vi "Motic Get Temperature.vi"(8 "error in (no error)":errorcluster, 11 "camera":i32) -> (0 "error out":errorcluster, 1 "ambient temperature out":sgl, 2 "sensor surface temperature out":sgl, 3 "camera out":i32, 4 "relative humidity out":sgl, 5 "is temperature data available?":bool)   [LabVIEW 2012, in "MoticApi.lvlib"]
doc: "MOTICAPI bool Motic_GetTemperature(MUCam_Handle camera, float* st, float*at, float*rh);"
uses:
  MoticApi.lvlib
  MoticApi.dll
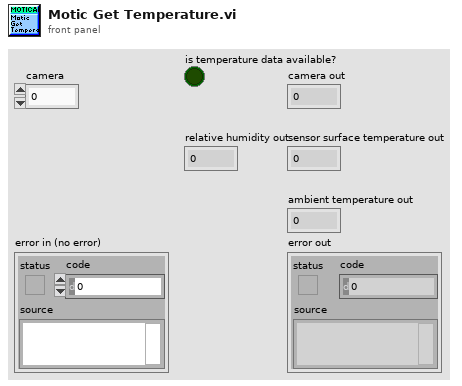
[diagram p1: front panel]
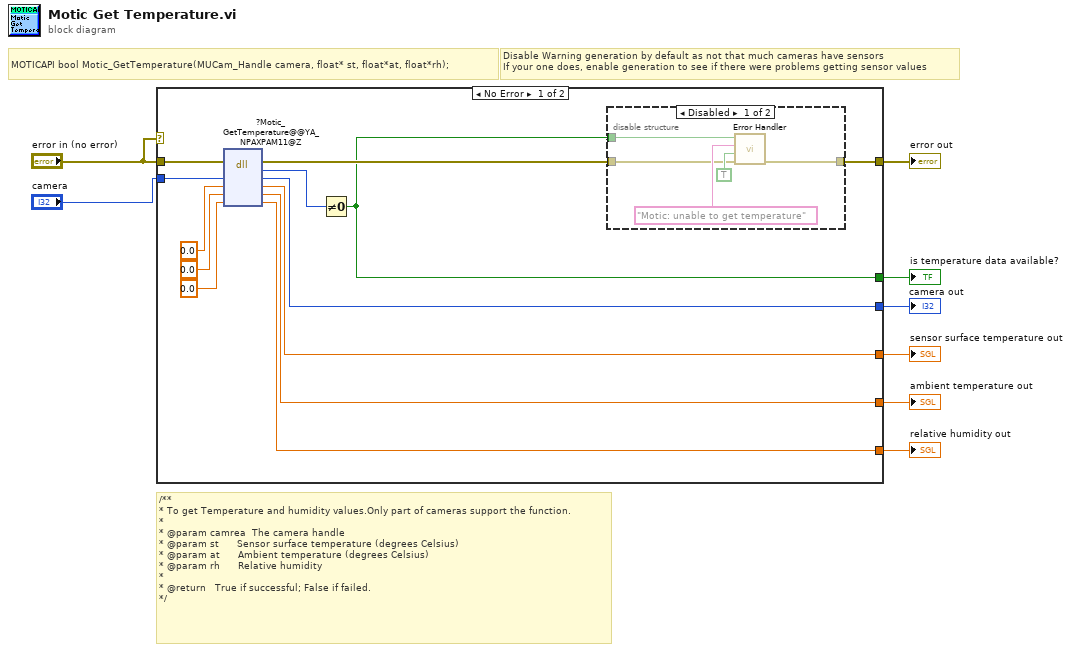
[diagram p0: block diagram]
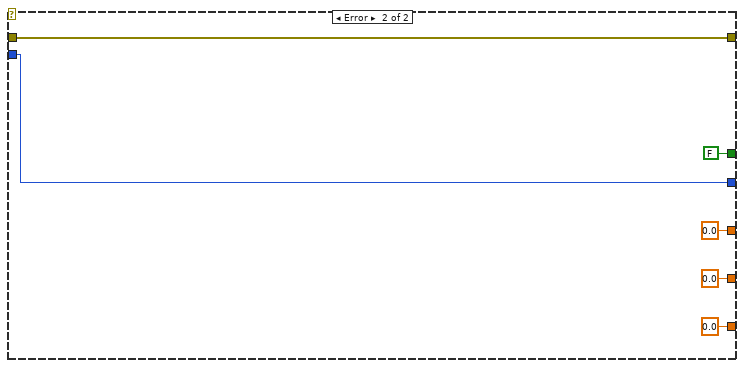
[diagram p3: hidden frame]
diagram:
  # "/**\n* To get Temperature and humidity values.Only part of cameras support the function.\n*\n* @param camrea  The camera handle\n* @param st      Sensor surface temperature (degrees Celsius)\n* @param at      Ambient temperature (degrees Celsius)\n* @param rh      Relative humidity\n*\n* @return   True if successful; False if failed.\n*/"
  # "Disable Warning generation by default as not that much cameras have sensors\nIf your one does, enable generation to see if there were problems getting sensor values"
  # "MOTICAPI bool Motic_GetTemperature(MUCam_Handle camera, float* st, float*at, float*rh);"
  n1 = case shown="No Error" "error in (no error)" {
    tunnel: "camera" -> [w20 w32]
    tunnel: [w18 sgl 0.0 ("st")] -> w7
    tunnel: [w16 sgl 0.0 ("at")] -> w6
    tunnel: [w14 sgl 0.0 ("rh")] -> w5
    tunnel: [w13 w33] -> w4
    tunnel: "error in (no error)" -> [w12 w33]
    tunnel: [w10 FALSE] -> w3
    tunnel: [w9 w32] -> w2
    frame No Error {
      n2 = dll-call lib="C:/Users/TTS-Digital/Desktop/MoticApi/MoticApi_git/MoticApi/MoticApi.*" fn="?Motic_GetTemperature@@YA_NPAXPAM11@Z"(error in=w12, "camera"=w20, "st"=sgl 0.0, "at"=sgl 0.0, "rh"=sgl 0.0) -> (error out=w11:errorcluster, "return type"=w21:u8, "camera"=w9:i32, "st"=w18:sgl, "at"=w16:sgl, "rh"=w14:sgl)  [unwired: 2 in, 1 out]
      n3 = Not Equal To 0?(x=w21) -> (x != 0?=w10:bool)
      n4 = disable-structure shown="Disabled" {
        disable-tunnel: [w24 w27] -> w13
        disable-tunnel: w11 -> [w23 w27]
        disable-tunnel: w10 -> [w22 _]
        frame Disabled {
          n5 = call "Error Handler.vi"("error in (no error)"=w23, "Is warning?"=TRUE, "Error message"="Motic: unable to get temperature", "Function return"=w22) -> ("error out"=w24:errorcluster)  [unwired: 7 in]
        }
        frame Enabled {
        }
      }
    }
    frame Error {
    }
  }
  "camera out" <- w2
  "sensor surface temperature out" <- w7
  "ambient temperature out" <- w6
  "relative humidity out" <- w5
  "error out" <- w4
  "is temperature data available?" <- w3
